vi "Main.vi"() -> ()   [LabVIEW 2013]
uses:
  System.Data
panel:
  out "Fehler (Ausgang)":errorcluster
  in  "Fehler (Eingang, kein Fehler)":errorcluster
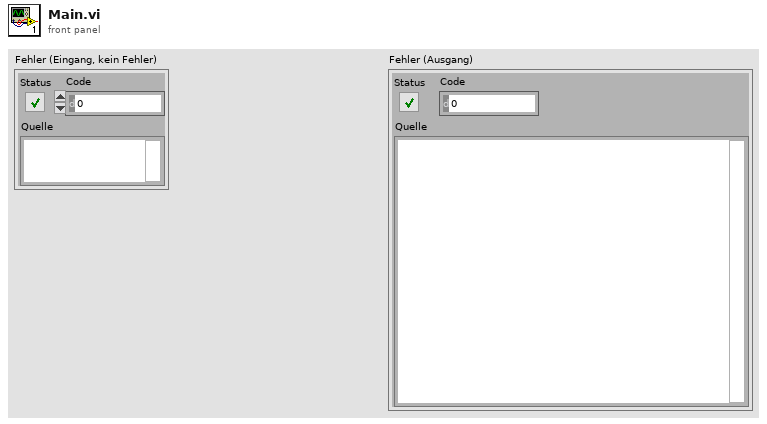
[diagram p1: front panel]
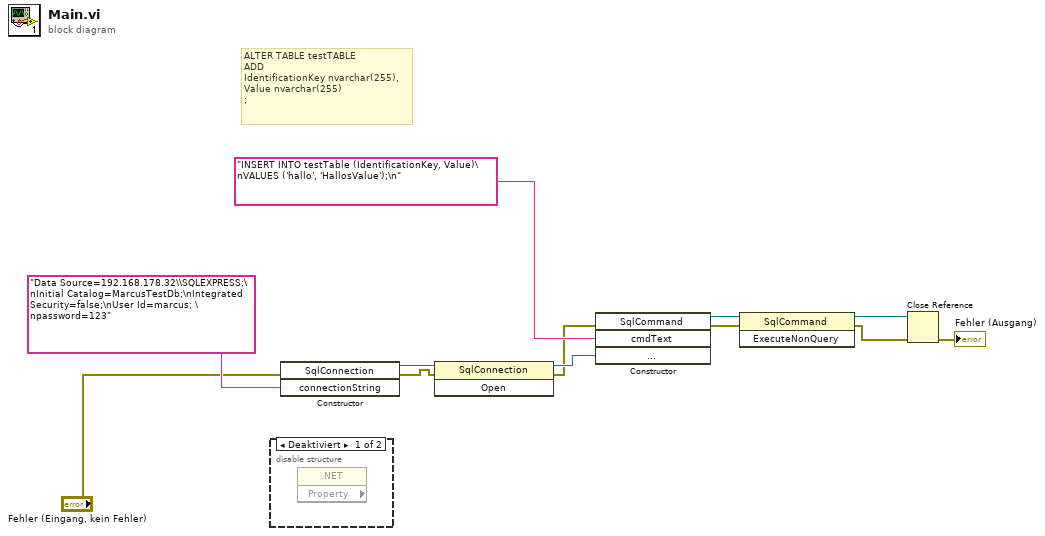
[diagram p0: block diagram]
diagram:
  # "ALTER TABLE testTABLE \nADD \nIdentificationKey nvarchar(255),\nValue nvarchar(255)\n;"
  n1 = disable-structure shown="Deaktiviert" {
    frame Disabled {
      n2 = property on="Eigenschaftsknoten" class=".NET" props=[]() -> ()  [unwired: 2 in, 3 out]
    }
    frame Enabled {
    }
  }
  n3 = constructor class="SqlConnection"(error in="Fehler (Eingang, kein Fehler)", "connectionString"="Data Source=192.168.178.32\\SQLEXPRESS;\nInitial Catalog=MarcusTestDb;\nIntegrated Security=false;\nUser Id=marcus; \npassword=123") -> (reference out=w11:refnum<k24>, error out=w9:errorcluster)  [unwired: 2 in, 2 out]
  n4 = invoke on="Methodenknoten" class="SqlConnection" method="Open"(reference=w11, error in=w9) -> (reference out=w7:refnum<k24>, error out=w5:errorcluster)  [unwired: 1 in, 1 out]
  n5 = constructor class="SqlCommand"(error in=w5, "cmdText"="INSERT INTO testTable (IdentificationKey, Value)\nVALUES ('hallo', 'HallosValue');\n", "connection"=w7) -> (reference out=w6:refnum<k24>, error out=w4:errorcluster)  [unwired: 2 in, 3 out]
  n6 = invoke class="SqlCommand" method="ExecuteNonQuery"(reference=w6, error in=w4) -> (reference out=w3:refnum<k24>, error out=w2:errorcluster)  [unwired: 1 in, 1 out]
  n7 = Close Reference(reference=w3, error in (no error)=w2) -> (error out=→"Fehler (Ausgang)":errorcluster)
